vi "SP Save Trace keys.vi"(6 "Trace":T1={"Trace On"=TRUE, "Measure"=0, "Format"=0, "Autoscale"=TRUE, "Reference"=0.0, "\nRefUnit"="dB/Div", "Position"=5.0, "Scale"=10.0, "ScaleUnit"="dB/Div", "LimitOn"=TRUE, "LimitFill"=FALSE, "Display Data"=0, "Show Markers"=TRUE, "SXX"=""} {"Reference" format="%#.2g"; "Display Data" items=["Data", "Memory", "Data/Memory"]; "Format" items=["Log Mag", "Phase", "Expanded Phase", "Delay", "Smith", "Polar", "Lin Mag", "SWR", "Loss", "Real", "Imaginary"]; "Scale" min=0.001 step=1.0 format="%#.2g"; "Position" min=0.0 max=10.0}, 7 "Prefix":string, 8 "error in (no error)":errorcluster, 9 "Channel Name In":string, 10 "Group Name In":string, 11 "TDMS File Ref In":refnum<k34>) -> (0 "error out":errorcluster, 1 "Channel Name Out":string, 2 "Group Name Out":string, 3 "TDMS File Ref Out":refnum<k34>)   [LabVIEW 2011]
uses:
  TypeDefs/SP Display Trace Controls.ctl
  TypeDefs/SP Display Format.ctl
  TypeDefs/SP Display Data.ctl
panel:
  # "Div"
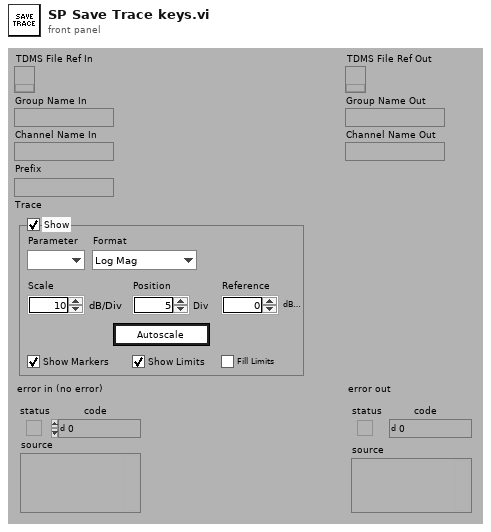
[diagram p1: front panel]
types:
  T1 = typedef "SP Display Trace Controls.ctl" = cluster{"Trace On":bool, "Measure":i32, "Format":T2, "Autoscale":bool, "Reference":dbl, "\nRefUnit":string, "Position":dbl, "Scale":dbl, "ScaleUnit":string, "LimitOn":bool, "LimitFill":bool, "Display Data":T3, "Show Markers":bool, "SXX":string}
  T2 = typedef "SP Display Format.ctl" = i32
  T3 = typedef "SP Display Data.ctl" = u16
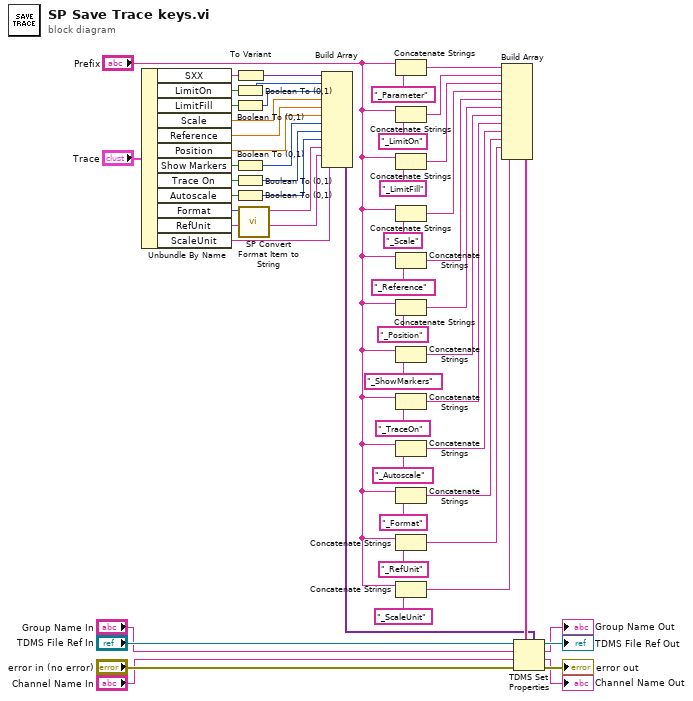
[diagram p0: block diagram]
diagram:
  n1 = Unbundle By Name("Trace") -> ("SXX"=w18:string, "LimitOn"=w51:bool, "LimitFill"=w50:bool, "Scale"=w9:dbl, "Reference"=w8:dbl, "Position"=w7:dbl, "Show Markers"=w39:bool, "Trace On"=w38:bool, "Autoscale"=w37:bool, "Format"=w19:T2, "RefUnit"=w2:string, "ScaleUnit"=w1:string)
  n2 = Boolean To (0,1)(Boolean=w51) -> (0, 1=w11:i16)
  n3 = Boolean To (0,1)(Boolean=w50) -> (0, 1=w10:i16)
  n4 = Boolean To (0,1)(Boolean=w39) -> (0, 1=w6:i16)
  n5 = Boolean To (0,1)(Boolean=w38) -> (0, 1=w5:i16)
  n6 = Boolean To (0,1)(Boolean=w37) -> (0, 1=w4:i16)
  n7 = To Variant(anything=w18) -> (Variant=w17:variant)
  n8 = call "SP Convert Format Item to String.vi"("Format"=w19) -> ("Format String"=w3:string)  [unwired: 6 out]
  n9 = Build Array(w17, w11, w10, w9, w8, w7, w6, w5, w4, w3, w2, w1) -> (w16:variant[])
  n10 = Concatenate Strings("Prefix", "_Parameter" ("sxFieldId")) -> (w32:string)
  n11 = Concatenate Strings("Prefix", "_LimitOn" ("sxFieldId")) -> (w31:string)
  n12 = Concatenate Strings("Prefix", "_LimitFill" ("sxFieldId")) -> (w30:string)
  n13 = Concatenate Strings("Prefix", "_Scale" ("sxFieldId")) -> (w29:string)
  n14 = Concatenate Strings("Prefix", "_Reference" ("sxFieldId")) -> (w28:string)
  n15 = Concatenate Strings("Prefix", "_Position" ("sxFieldId")) -> (w27:string)
  n16 = Concatenate Strings("Prefix", "_ShowMarkers" ("sxFieldId")) -> (w26:string)
  n17 = Concatenate Strings("Prefix", "_TraceOn" ("sxFieldId")) -> (w25:string)
  n18 = Concatenate Strings("Prefix", "_Autoscale" ("sxFieldId")) -> (w24:string)
  n19 = Concatenate Strings("Prefix", "_Format" ("sxFieldId")) -> (w23:string)
  n20 = Concatenate Strings("Prefix", "_RefUnit" ("sxFieldId")) -> (w22:string)
  n21 = Concatenate Strings("Prefix", "_ScaleUnit" ("sxFieldId")) -> (w21:string)
  n22 = Build Array(w32, w31, w30, w29, w28, w27, w26, w25, w24, w23, w22, w21) -> (w20:string[])
  n23 = TDMS Set Properties(5:w16, 7:w20, 8:"error in (no error)", 9:"Channel Name In", 10:"Group Name In", 11:"TDMS File Ref In") -> (0:→"error out":errorcluster, 1:→"Channel Name Out":string, 2:→"Group Name Out":string, 3:→"TDMS File Ref Out":refnum<k34>)
